vi "Send SPI Engine Response 128-bit.vi"(8 "error in":errorcluster, 9 "Input Valid":bool, 10 "Response Data":T1, 11 "SPI Engine Resources":T3={"To SPI Engine Data FIFO"="DLU To SPI Engine Data FIFO", "From SPI Engine Data FIFO"="SPI Engine to DLU Data FIFO", "Data to SPI Engine Cache Register"="Data to SPI Engine (Cache)", "SPI Transaction Settings Cache Register"="SPI PHY Settings to SPI Engine (Cache)"}) -> (0 "error out":errorcluster, 1 "New Data Sent?":bool, 2 "Response Data":T1, 3 "SPI Engine Resources":T3={"To SPI Engine Data FIFO"="DLU To SPI Engine Data FIFO", "From SPI Engine Data FIFO"="SPI Engine to DLU Data FIFO", "Data to SPI Engine Cache Register"="Data to SPI Engine (Cache)", "SPI Transaction Settings Cache Register"="SPI PHY Settings to SPI Engine (Cache)"}, 4 "Ready for Input":bool)   [LabVIEW 2015, in "SPI API.lvlib"]
doc: "This VI conditionally writes new data to the SPI Response FIFO."
uses:
  SPI API.lvlib
  Controls/SPI Engine Resources 128-bit.ctl
  Controls/SPI API Response Data 128-bit.ctl
  Controls/SPI API Data 128-bit.ctl
  SPI Engine.Send Response Data.Write FIFO 128-bit.vi
panel:
  out "Data Sent First":T1
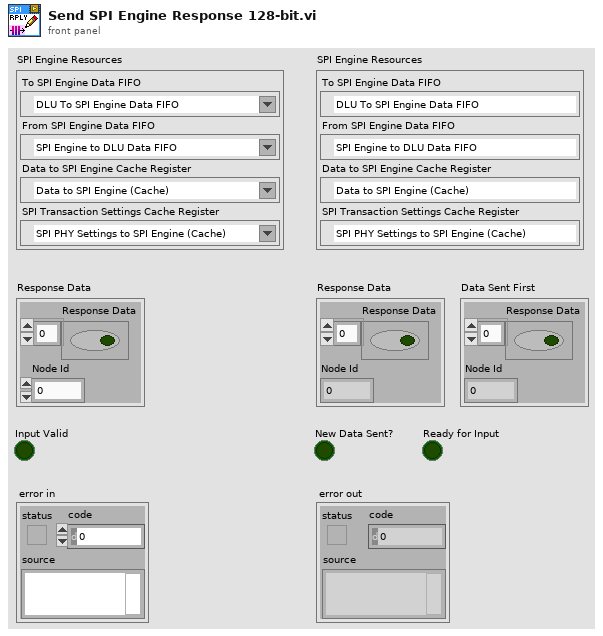
[diagram p1: front panel]
types:
  T1 = typedef "SPI API.lvlib/SPI API Response Data 128-bit.ctl" = cluster{"Response Data":T2, "Node Id":u16}
  T2 = typedef "SPI API.lvlib/SPI API Data 128-bit.ctl" = bool[]
  T3 = typedef "SPI API.lvlib/SPI Engine Resources 128-bit.ctl" = cluster{"To SPI Engine Data FIFO":refnum<k21>, "From SPI Engine Data FIFO":refnum<k21>, "Data to SPI Engine Cache Register":refnum<k21>, "SPI Transaction Settings Cache Register":refnum<k21>}
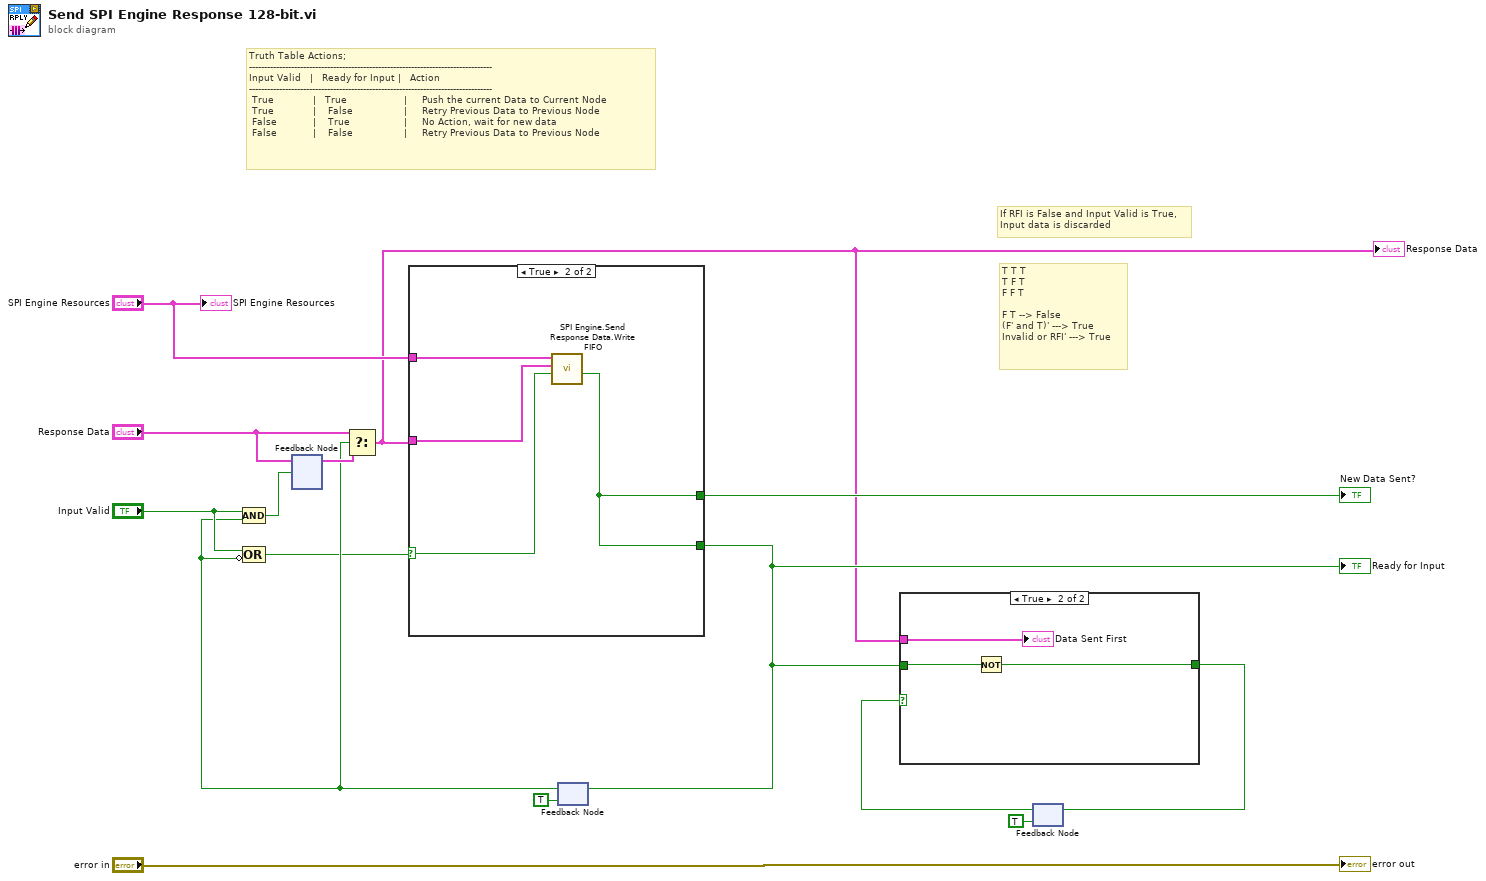
[diagram p0: block diagram]
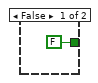
[diagram p2: hidden frame]
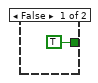
[diagram p3: hidden frame]
diagram:
  # "T T T\nT F T\nF F T\n\nF T --> False\n(F' and T)' ---> True\nInvalid or RFI' ---> True"
  # "If RFI is False and Input Valid is True,\nInput data is discarded"
  # "Truth Table Actions;\n---------------------------------------------------------------------------------\nInput Valid   |   Ready for Input |   Action\n---------------------------------------------------------------------------------\n True             |   True                   |     Push the current Data to Current Node\n True             |    False                 |     Retry Previous Data to Previous Node\n False            |    True                  |     No Action, wait for new data\n False            |    False                 |     Retry Previous Data to Previous Node"
  n1 = feedback #1() -> (w12:T1)  [unwired: 1 in]
  n2 = feedback #2(TRUE ("Send Success?")) -> (w9:bool)
  n3 = Compound Arithmetic op=AND("Input Valid", w9) -> (w14:bool)
  n4 = Compound Arithmetic op=OR("Input Valid", invert w9) -> (w8:bool)
  n5 = feedback-in #1("Response Data", w14) -> ()
  n6 = Select(t="Response Data", s=w9, f=w12) -> (s? t:f=w1:T1)
  "Response Data" <- w1
  n7 = case shown="True" w8 {
    selector: w8 -> [_ w18]
    tunnel: "SPI Engine Resources" -> [_ w20]
    tunnel: w1 -> [_ w19]
    tunnel: [TRUE ("Send Success?") w17] -> w7
    tunnel: [_ w17] -> w10
    frame False {
    }
    frame True {
      n8 = call-poly "SPI Engine.Send Response Data.Write FIFO.vi"("Input Valid"=w18, "Response Data"=w19, "SPI Engine Resources"=w20) -> ("Send Success?"=w17:bool)  [unwired: 6 in, 2 out]
    }
  }
  "Ready for Input" <- w7
  "New Data Sent?" <- w10
  n9 = feedback-in #2(w7) -> ()
  n10 = feedback #3(TRUE) -> (w5:bool)
  n11 = case shown="True" w5 {
    tunnel: w1 -> [_ w22]
    tunnel: w7 -> [_ w24]
    tunnel: [FALSE w23] -> w6
    frame False {
    }
    frame True {
      n12 = Not(x=w24) -> (.not. x?=w23:bool)
      "Data Sent First" <- w22
    }
  }
  n13 = feedback-in #3(w6) -> ()
  "error out" <- "error in"
  "SPI Engine Resources" <- "SPI Engine Resources"
